vi "Unmute.vi"(7 "Direction":T1, 8 "error in (no error)":errorcluster, 10 "Index":i32, 11 "VoiceMeeterRemote in":refnum<class "VoiceMeeterRemote.lvclass">) -> (0 "error out":errorcluster, 3 "VoiceMeeterRemote out":refnum<class "VoiceMeeterRemote.lvclass">)   [LabVIEW 2022 SP3, in "VoiceMeeterRemote.lvlib" / "VoiceMeeterRemote.lvclass"]
doc: "Unmutes the specified input or output index."
uses:
  VoiceMeeterRemote.lvclass
  Direction.ctl
  VoiceMeeterRemote.lvlib
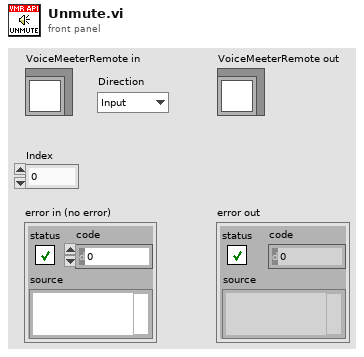
[diagram p1: front panel]
types:
  T1 = typedef "VoiceMeeterRemote.lvlib/Direction.ctl" = enum16{"Input", "Output"}
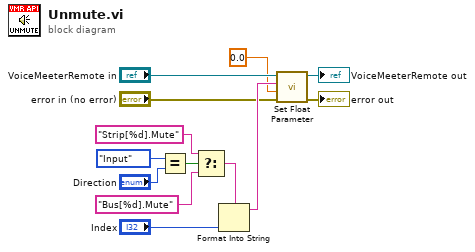
[diagram p0: block diagram]
diagram:
  n1 = Equal?(x=Direction."Input", y="Direction") -> (x = y?=w11:bool)
  n2 = Select(t="Strip[%d].Mute", s=w11, f="Bus[%d].Mute") -> (s? t:f=w8:string)
  n3 = Format Into String(format string=w8, "Index") -> (resulting string=w5:string)  [unwired: 2 in, 1 out]
  n4 = call "Set Float Parameter.vi"("error in (no error)"="error in (no error)", "Value"=sgl 0.0, "Parameter Name"=w5, "VoiceMeeterRemote in"="VoiceMeeterRemote in") -> ("error out"=→"error out":errorcluster, "VoiceMeeterRemote out"=→"VoiceMeeterRemote out":refnum<class "VoiceMeeterRemote.lvclass">)  [unwired: 6 in]
